vi "COL INDEX SWITCH.vi"(10 "INDEX":T1, 11 "NM?":bool) -> (0 "col etag":i32, 1 "col P2":i32, 2 "col NPSH":i32, 3 "col Htot":i32, 5 "col Q":i32)   [LabVIEW 2019]
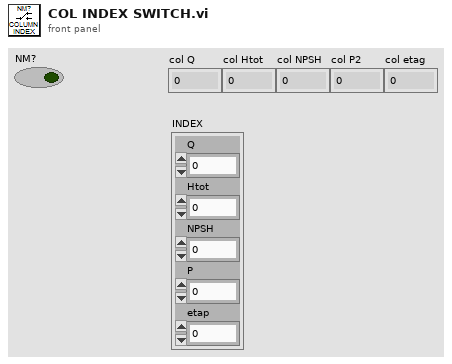
[diagram p1: front panel]
types:
  T1 = cluster{"Q":i32, "Htot":i32, "NPSH":i32, "P":i32, "etap":i32}
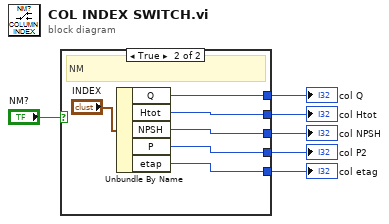
[diagram p0: block diagram]
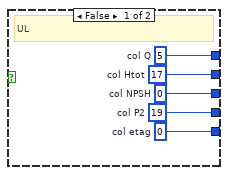
[diagram p2: hidden frame]
diagram:
  n1 = case shown="True" "NM?" {
    tunnel: [w11 w16] -> w2
    tunnel: [w10 w15] -> w3
    tunnel: [w9 w14] -> w4
    tunnel: [w8 w13] -> w5
    tunnel: [w7 w12] -> w6
    frame False {
      w7 = 0  # col etag
      w8 = 19  # col P2
      w9 = 0  # col NPSH
      w10 = 17  # col Htot
      w11 = 5  # col Q
      # "UL"
    }
    frame True {
      # "NM"
      n2 = Unbundle By Name("INDEX") -> ("Q"=w16:i32, "Htot"=w15:i32, "NPSH"=w14:i32, "P"=w13:i32, "etap"=w12:i32)
    }
  }
  "col etag" <- w6
  "col P2" <- w5
  "col NPSH" <- w4
  "col Htot" <- w3
  "col Q" <- w2
